vi "Test Animal Can Eat after Sleeping.vi"(8 "error in (no error)":errorcluster, 11 "Animal Test In":refnum<class "Animal Test.lvclass">) -> (0 "error out":errorcluster, 3 "Animal Test Out":refnum<class "Animal Test.lvclass">)   [LabVIEW 2020, in "Animal Test.lvclass"]
doc: "Test Animal can eat after sleeping."
uses:
  Animal Test.lvclass
  C:/Program Files (x86)/National Instruments/LabVIEW 2020/vi.lib/Astemes/LUnit/Test Case.lvclass
  Animal Test.lvclass/Animal Test.ctl
  <vilib>/Astemes/LUnit/Test Case.lvclass/Test Case.ctl
  e54b3c1c-751e-47bd-9c9d-03426323aa40.vi
  <vilib>/Astemes/LUnit/Append Pass Result.vi
  <vilib>/Astemes/LUnit/Append Fail Result.vi
  <vilib>/Astemes/LUnit/Describe Comparison.vi
  <vilib>/Astemes/LUnit/Compare Variants.vi
  <vilib>/Astemes/LUnit/Run In UI.vi
  <vilib>/Utility/error.llb/Clear Errors.vi
  <vilib>/Astemes/LUnit/Describe Variant.vi
  Animal Classes/Animal/Animal.lvclass
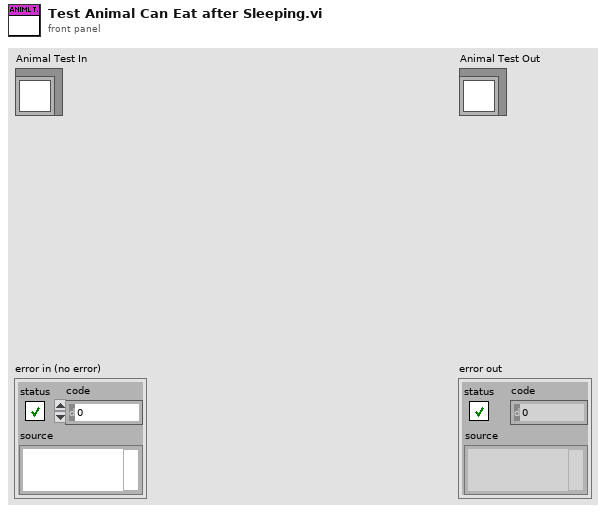
[diagram p1: front panel]
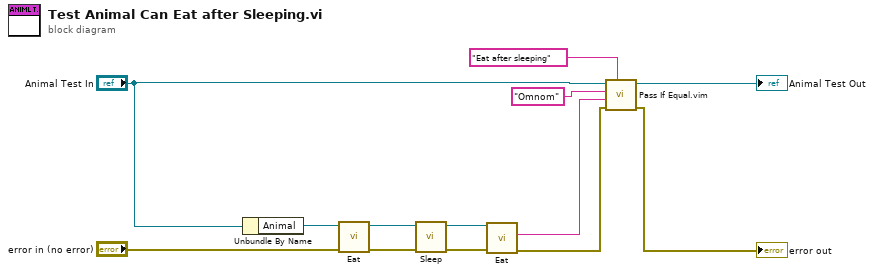
[diagram p0: block diagram]
diagram:
  n1 = Unbundle By Name("Animal Test In") -> ("Animal"=w11:refnum<class "Animal.lvclass">)
  n2 = call-dynamic "Eat.vi"("error in (no error)"="error in (no error)", "Animal In"=w11) -> ("error out"=w12:errorcluster, "Animal Out"=w13:refnum<class "Animal.lvclass">)  [unwired: 7 in, 1 out]
  n3 = call-dynamic "Sleep.vi"("error in (no error)"=w12, "Animal in"=w13) -> ("error out"=w7:errorcluster, "Animal out"=w10:refnum<class "Animal.lvclass">)  [unwired: 7 in, 1 out]
  n4 = call-dynamic "Eat.vi"("error in (no error)"=w7, "Animal In"=w10) -> ("error out"=w2:errorcluster, "Result"=w3:string)  [unwired: 7 in, 1 out]
  n5 = call "Pass If Equal.vim"("Description"="Eat after sleeping", "error in (no error)"=w2, "Actual"=w3, "Expected"="Omnom" ("Description"), "LUnit Test Case In"="Animal Test In") -> ("error out"=→"error out":errorcluster, "LUnit Test Case Out"=→"Animal Test Out":refnum<class "Animal Test.lvclass">)  [unwired: 5 in]
